vi "ExportAgingDataToExcel.vi"(1 "AgingData":string[][](array[string])=array13108x3[39324 elements], 2 "HeaderAging":string[](array[string])=["time (h)", "P (mW/cm2)", " "], 3 "DeviceNames":string[](array[string])=["Ch5_Device5"], 4 "JVMetricsData":string[][](array[string])=[["2.233623E-4", "2.809920E-4", "1.250938E-1", "1.296342E-4", "1.732760E+1", "9.119407E-1", ""], ["5.130579E-1", "1.862739E-4", "7.606130E-1", "1.251912E-4", "1.956205E+0", "5.641287E-1", ""], ["1.021197E+0", "3.139945E-4", "3.830989E-1", "1.999200E-4", "4.099727E+0", "6.239515E-1", ""], ["1.529947E+0", "3.112586E-4", "-1.422943E-1", "-2.189960E-4", "9.988443E+0", "5.569672E-1", ""], ["2.038474E+0", "6.684978E-4", "6.387401E-1", "-1.152281E-4", "-9.082747E+0", "7.913465E-1", ""], ["2.547363E+0", "2.737201E-4", "3.765440E-1", "2.384102E-4", "3.049062E+0", "5.665012E-1", ""], ["3.056419E+0", "3.429767E-4", "1.047323E-1", "5.488136E-4", "5.967041E+0", "6.079894E-1", ""], ["3.566641E+0", "2.248290E-4", "4.767564E-1", "-6.361813E-5", "-7.412673E+0", "9.647748E-1", ""], ["4.079095E+0", "3.226346E-4", "7.726537E-1", "-4.322167E-4", "-9.661053E-1", "6.524026E-1", ""], ["4.588696E+0", "3.433145E-4", "4.112062E-1", "1.872766E-5", "4.458092E+1", "9.480473E-1", ""], ["5.098863E+0", "3.364492E-4", "7.053339E-1", "-3.665195E-4", "-1.301450E+0", "1.121436E+0", ""], ["5.611697E+0", "7.171495E-4", "-3.941252E-2", "2.893143E-4", "-6.289349E+1", "2.199100E+0", ""], ["6.123613E+0", "4.661567E-4", "6.952749E-1", "-1.136010E-4", "-5.901919E+0", "6.618966E-1", ""], ["6.639169E+0", "5.280098E-4", "4.587868E-1", "-2.428356E-5", "-4.739350E+1", "1.288842E+0", ""], ["7.153391E+0", "1.963873E-4", "2.158962E-1", "-3.646201E-4", "-2.494754E+0", "5.255405E-1", ""], ["7.666752E+0", "3.913245E-4", "1.911950E-1", "-1.876979E-4", "-1.090439E+1", "9.657755E-1", ""], ["8.187641E+0", "4.770075E-4", "3.844965E-1", "5.572484E-4", "2.226301E+0", "9.086906E-1", ""], ["8.708586E+0", "2.176574E-4", "1.495751E-1", "-2.121337E-4", "-6.859688E+0", "5.325443E-1", ""], ["9.221725E+0", "2.481350E-4", "7.114364E-1", "1.472181E-4", "2.369139E+0", "7.226222E-1", ""], ["9.739197E+0", "6.917812E-4", "2.285220E-1", "-3.087242E-5", "-9.805506E+1", "1.335809E+0", ""], ["1.025436E+1", "4.406193E-4", "5.324292E-1", "8.008906E-5", "1.033305E+1", "2.150808E+0", ""], ["1.077695E+1", "4.729752E-4", "3.706222E-1", "-1.765112E-4", "-7.229941E+0", "1.440072E+0", ""], ["1.129897E+1", "3.317154E-4", "8.815467E-1", "-3.532666E-4", "-1.065167E+0", "1.099985E+0", ""], ["1.182495E+1", "1.625717E-4", "3.648582E-1", "9.818597E-6", "4.538071E+1", "4.985518E-1", ""], ["1.235353E+1", "3.655197E-4", "-7.214136E-2", "1.764439E-4", "-2.871573E+1", "8.038818E-1", ""], ["1.289901E+1", "1.485624E-4", "2.690905E-1", "-3.835743E-4", "-1.439332E+0", "3.139778E-1", ""], ["1.343053E+1", "3.381395E-4", "5.715721E-1", "2.136598E-4", "2.768866E+0", "1.188202E+0", ""], ["1.395144E+1", "2.392585E-4", "1.248513E-2", "1.785137E-4", "1.073502E+2", "1.047871E+0", ""]]) -> ()   [LabVIEW 2020]
uses:
  <vilib>/Utility/NIReport.llb/NI_report.lvclass
  <vilib>/addons/_office/excel.llb/Excel Easy Table (str).vi
panel:
  in  "HeaderJVMetrics":string[](array[string])=["time (h)", "Voc (V)", "Jsc (mA/cm2)", "FF", "P (mW/cm2)", "Hyst (P1/P2)", "  "]
  out "Worksheet Index":i32=1
  in  "title":string="AgingExport "
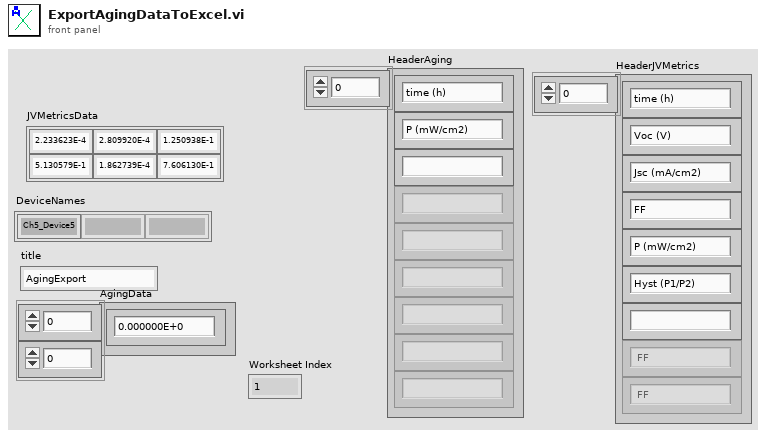
[diagram p1: front panel]
types:
  T1 = enum16{"Standard Report", "HTML", "Word", "Excel"}
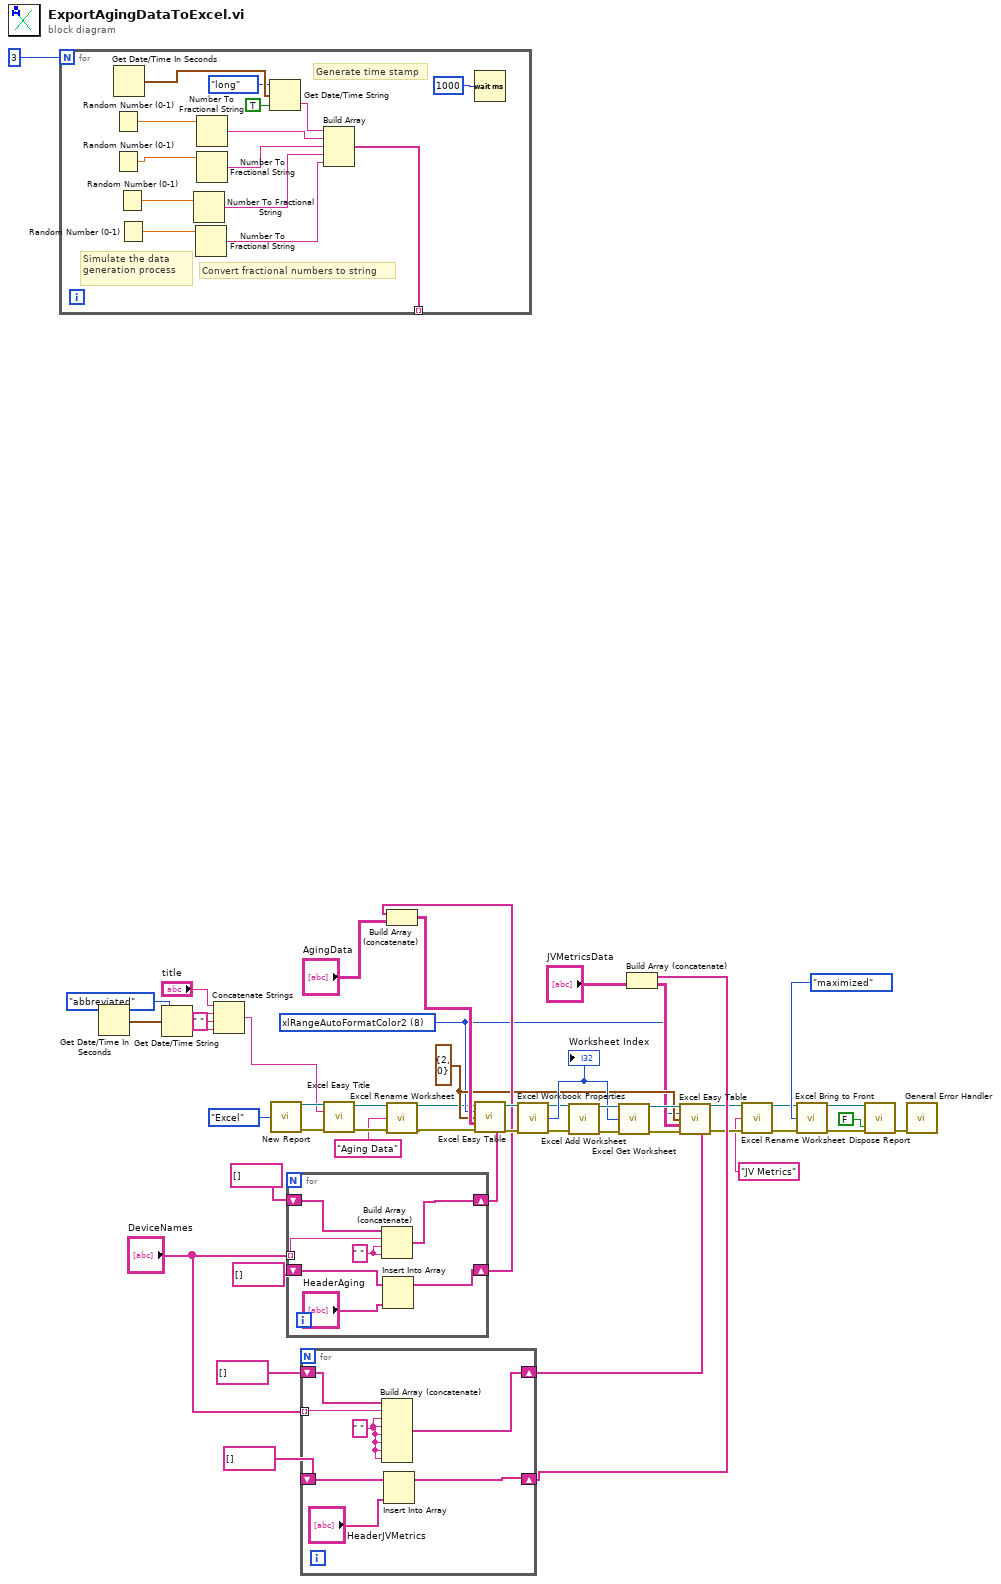
[diagram p0: block diagram]
diagram:
  w11 = 8 items=["xlRangeAutoFormat3DEffects1"=13, "xlRangeAutoFormat3DEffects2"=14, "xlRangeAutoFormatAccounting1"=4, "xlRangeAutoFormatAccounting2"=5, "xlRangeAutoFormatAccounting3"=6, "xlRangeAutoFormatAccounting4"=17, "xlRangeAutoFormatClassic1"=1, "xlRangeAutoFormatClassic2"=2, "xlRangeAutoFormatClassic3"=3, "xlRangeAutoFormatColor1"=7, "xlRangeAutoFormatColor2"=8, "xlRangeAutoFormatColor3"=9, "xlRangeAutoFormatList1"=10, "xlRangeAutoFormatList2"=11, "xlRangeAutoFormatList3"=12, "xlRangeAutoFormatLocalFormat1"=15, "xlRangeAutoFormatLocalFormat2"=16, "xlRangeAutoFormatLocalFormat3"=19, "xlRangeAutoFormatLocalFormat4"=20, "xlRangeAutoFormatReport1"=21, "xlRangeAutoFormatReport2"=22, "xlRangeAutoFormatReport3"=23, "xlRangeAutoFormatReport4"=24, "xlRangeAutoFormatReport5"=25, "xlRangeAutoFormatReport6"=26, "xlRangeAutoFormatReport7"=27, "xlRangeAutoFormatReport8"=28, "xlRangeAutoFormatReport9"=29, "xlRangeAutoFormatReport10"=30, "xlRangeAutoFormatClassicPivotTable"=31, "xlRangeAutoFormatTable1"=32, "xlRangeAutoFormatTable2"=33, "xlRangeAutoFormatTable3"=34, "xlRangeAutoFormatTable4"=35, "xlRangeAutoFormatTable5"=36, "xlRangeAutoFormatTable6"=37, "xlRangeAutoFormatTable7"=38, "xlRangeAutoFormatTable8"=39, "xlRangeAutoFormatTable9"=40, "xlRangeAutoFormatTable10"=41, "xlRangeAutoFormatPTNone"=42, "xlRangeAutoFormatNone"=-4142, "xlRangeAutoFormatSimple"=-4154] ("auto format")
  w15 = cluster{"row":i32, "column":i32} {"row"=2, "column"=0} ("position")
  n1 = for {
    N: 3 -> [_]
    tunnel: [w53] -> _ mode=indexing
    # "Convert fractional numbers to string"
    # "Generate time stamp"
    # "Simulate the data generation process"
    n2 = Random Number (0-1)() -> (number: 0 to 1=w61:dbl)
    n3 = Random Number (0-1)() -> (number: 0 to 1=w60:dbl)
    n4 = Get Date/Time In Seconds() -> (seconds since 1Jan1904=w64:timestamp)
    n5 = Random Number (0-1)() -> (number: 0 to 1=w59:dbl)
    n6 = Random Number (0-1)() -> (number: 0 to 1=w58:dbl)
    n7 = Number To Fractional String(number=w59) -> (F-format string=w55:string)  [unwired: 3 in]
    n8 = Number To Fractional String(number=w58) -> (F-format string=w54:string)  [unwired: 3 in]
    n9 = Number To Fractional String(number=w61) -> (F-format string=w57:string)  [unwired: 3 in]
    n10 = Number To Fractional String(number=w60) -> (F-format string=w56:string)  [unwired: 3 in]
    n11 = Get Date/Time String(date format (0)=enum16{"short", "long", "abbreviated"}."long", seconds (now)=w64, want seconds? (F)=TRUE) -> (time string=w51:string)  [unwired: 1 out]
    n12 = Build Array(w51, w57, w56, w55, w54) -> (w53:string[])
    n13 = Wait (ms)(milliseconds to wait=u32 1000) -> ()  [unwired: 1 out]
  }
  n14 = Get Date/Time In Seconds() -> (seconds since 1Jan1904=w39:timestamp)
  n15 = Get Date/Time String(date format (0)=enum16{"short", "long", "abbreviated"}."abbreviated", seconds (now)=w39) -> (date string=w38:string, time string=w36:string)  [unwired: 1 in]
  n16 = Concatenate Strings("title", w38, " " ("string"), w36) -> (w34:string)
  n17 = call <vilib>:"New Report.vi"("report type"=T1."Excel") -> ("report out"=w47:refnum<class "NI_report.lvclass">, "error out"=w48:errorcluster)  [unwired: 13 in]
  n18 = for {
    tunnel: "DeviceNames" -> [w70] mode=indexing
    shift-right: [w69] -> w31
    shift-left: string[] [] -> [w68]
    shift-right: [w67] -> w16
    shift-left: string[] [] -> [w66]
    w71 = " " ("element")
    n19 = Build Array (concatenate)(w68, w70, w71, w71) -> (w69:string[])
    n20 = Insert Into Array(array=w66, new element="HeaderAging") -> (w67:string[])  [unwired: 1 in]
  }
  n21 = for {
    tunnel: "DeviceNames" -> [w78] mode=indexing
    shift-right: [w75] -> w28
    shift-left: string[] [] -> [w77]
    shift-right: [w74] -> w12
    shift-left: string[] [] -> [w73]
    w76 = " " ("element")
    n22 = Build Array (concatenate)(w77, w78, w76, w76, w76, w76, w76, w76) -> (w75:string[])
    n23 = Insert Into Array(array=w73, new element="HeaderJVMetrics") -> (w74:string[])  [unwired: 1 in]
  }
  n24 = call <vilib>:"Excel Easy Title.vi"("report in"=w47, "title"=w34, "error in (no error)"=w48) -> ("report out"=w5:refnum<class "NI_report.lvclass">, "error out"=w2:errorcluster)  [unwired: 10 in, 1 out]
  n25 = Build Array (concatenate)(w16, "AgingData") -> (w41:string[][])
  n26 = call <vilib>:"Excel Rename Worksheet.vi"("report in"=w5, "worksheet name (\"\")"="Aging Data" ("name (\"\")"), "error in (no error)"=w2) -> ("report out"=w4:refnum<class "NI_report.lvclass">, "error out"=w3:errorcluster)  [unwired: 11 in]
  n27 = call-poly <vilib>:"Excel Easy Table.vi"("report in"=w4, "auto format (none)"=w11, "start (0, 0)"=w15, "text data"=w41, "error in (no error)"=w3, "column headers"=w31) -> ("report out"=w19:refnum<class "NI_report.lvclass">, "error out"=w20:errorcluster)  [unwired: 5 in, 3 out]
  n28 = call <vilib>:"Excel Workbook Properties.vi"("report in"=w19, "error in (no error)"=w20) -> ("report out"=w23:refnum<class "NI_report.lvclass">, "worksheets count"=w25:i32, "error out"=w24:errorcluster)  [unwired: 10 in, 1 out]
  "Worksheet Index" <- w25
  n29 = call <vilib>:"Excel Add Worksheet.vi"("report in"=w23, "error in (no error)"=w24) -> ("report out"=w26:refnum<class "NI_report.lvclass">, "error out"=w27:errorcluster)  [unwired: 12 in]
  n30 = call <vilib>:"Excel Get Worksheet.vi"("report in"=w26, "worksheet index (0)"=w25, "error in (no error)"=w27) -> ("report out"=w22:refnum<class "NI_report.lvclass">, "error out"=w21:errorcluster)  [unwired: 11 out]
  n31 = Build Array (concatenate)(w12, "JVMetricsData") -> (w14:string[][])
  n32 = call-poly <vilib>:"Excel Easy Table.vi"("report in"=w22, "auto format (none)"=w11, "start (0, 0)"=w15, "text data"=w14, "error in (no error)"=w21, "column headers"=w28) -> ("report out"=w9:refnum<class "NI_report.lvclass">, "error out"=w8:errorcluster)  [unwired: 5 in, 3 out]
  n33 = call <vilib>:"Excel Rename Worksheet.vi"("report in"=w9, "worksheet name (\"\")"="JV Metrics" ("worksheet name (\"\")"), "error in (no error)"=w8) -> ("report out"=w10:refnum<class "NI_report.lvclass">, "error out"=w7:errorcluster)  [unwired: 11 in]
  n34 = call <vilib>:"Excel Bring to Front.vi"("report in"=w10, "window state (maximized)"=enum16{"maximized", "minimized", "normal"}."maximized", "error in (no error)"=w7) -> ("report out"=w44:refnum<class "NI_report.lvclass">, "error out"=w45:errorcluster)  [unwired: 11 in]
  n35 = call-dynamic "Dispose Report.vi"("report in"=w44, "error in (no error)"=w45, "close report? (T)"=FALSE ("Close Report? (T)")) -> ("error out"=w43:errorcluster)  [unwired: 12 in]
  n36 = call <vilib>:"General Error Handler.vi"("error in (no error)"=w43) -> ()  [unwired: 10 in, 5 out]
